vi "LVLibNameFromFileName.vi"(11 "VI Name / CTL Name / LVCLASS Name":string) -> (3 "Library Name":string)   [LabVIEW 2019, in "Hawkeye.lvlib"]
uses:
  Hawkeye.lvlib
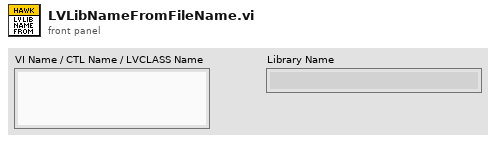
[diagram p1: front panel]
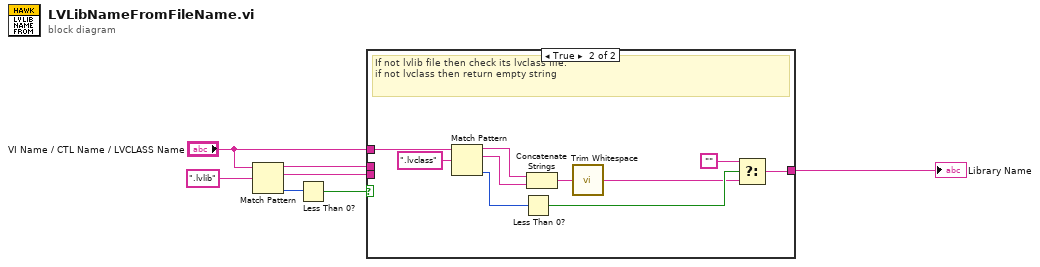
[diagram p0: block diagram]
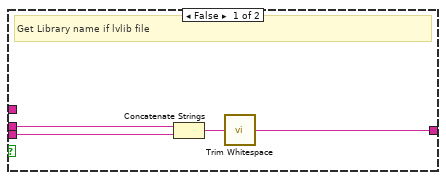
[diagram p2: hidden frame]
diagram:
  n1 = Match Pattern(string="VI Name / CTL Name / LVCLASS Name", regular expression=".lvlib") -> (before substring=w6:string, match substring=w5:string, offset past match=w3:i32)  [unwired: 1 in, 1 out]
  n2 = Less Than 0?(x=w3) -> (x < 0?=w2:bool)
  n3 = case shown="True" w2 {
    tunnel: w6 -> [w11 _]
    tunnel: w5 -> [w10 _]
    tunnel: [w8 w14] -> w4
    tunnel: "VI Name / CTL Name / LVCLASS Name" -> [_ w21]
    frame False {
      # "Get Library name if lvlib file"
      n4 = Concatenate Strings(w11, w10) -> (w9:string)
      n5 = call <vilib>:"Trim Whitespace.vi"("string"=w9) -> ("trimmed string"=w8:string)  [unwired: 1 in]
    }
    frame True {
      # "If not lvlib file then check its lvclass file.\nif not lvclass then return empty string"
      n6 = Match Pattern(string=w21, regular expression=".lvclass") -> (before substring=w12:string, match substring=w13:string, offset past match=w18:i32)  [unwired: 1 in, 1 out]
      n7 = Less Than 0?(x=w18) -> (x < 0?=w17:bool)
      n8 = Concatenate Strings(w12, w13) -> (w19:string)
      n9 = call <vilib>:"Trim Whitespace.vi"("string"=w19) -> ("trimmed string"=w16:string)  [unwired: 1 in]
      n10 = Select(t="" ("trimmed string"), s=w17, f=w16) -> (s? t:f=w14:string)
    }
  }
  "Library Name" <- w4
